vi "Do Core.vi"(8 "error in (no error)":errorcluster, 9 "Actor in":refnum<class "Actor.lvclass">, 11 "Reply Message":refnum<class "Init Msg.lvclass">) -> (0 "error out":errorcluster, 1 "Actor out":refnum<class "Actor.lvclass">, 2 "Reply":variant)   [LabVIEW 2022 SP3, in "ImageHandler.lvlib" / "Init Msg.lvclass"]
doc: "(<B>Filename</B>: Actor Framework.lvlib:Reply Msg.lvclass:Do Core.vi)\n\nDefines what an actor does when it receives <B>Reply Message</B>. This method also defines the <B>Reply</B> that is returned to the actor that sent <B>Reply Message</B>.\n\nBy default, this method does nothing, and <B>Reply</B> is the ancestor Message class. A child class must override this method to define behavior and specify a child of the Message class to return in the <B>Reply</B> output."
uses:
  <vilib>/ActorFramework/Actor/Actor.lvclass
  Init Msg.lvclass
  Init Msg.lvclass/Init Msg.ctl
  <vilib>/ActorFramework/Reply Msg/Reply Msg.lvclass
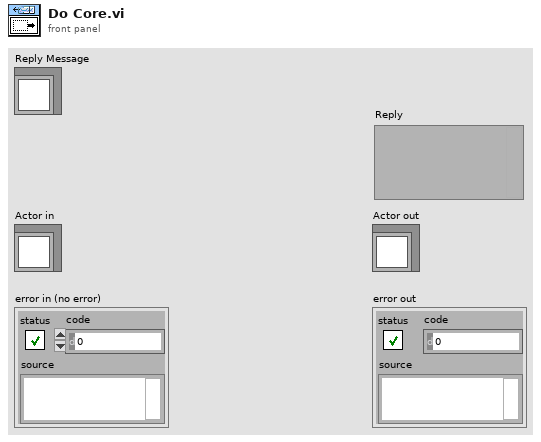
[diagram p1: front panel]
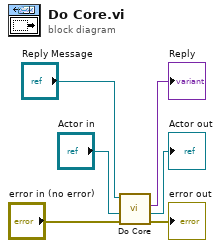
[diagram p0: block diagram]
diagram:
  n1 = call-parent "Do Core.vi"("error in (no error)"="error in (no error)", "Actor in"="Actor in", "Reply Message"="Reply Message") -> ("error out"=→"error out":errorcluster, "Actor out"=→"Actor out":refnum<class "Actor.lvclass">, "Reply"=→"Reply":variant)  [unwired: 6 in]
